vi "Construct LV Version String.vi"(8 "error in (no error)":errorcluster) -> (0 "error out":errorcluster, 3 "LabVIEW Version":string)   [LabVIEW 2014]
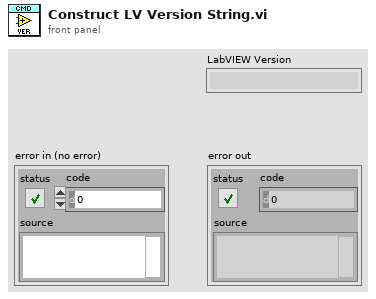
[diagram p1: front panel]
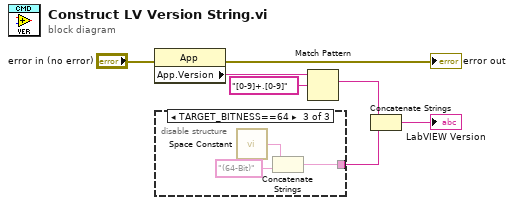
[diagram p0: block diagram]
diagram:
  n1 = property class="App"(error in="error in (no error)") -> (error out=→"error out":errorcluster, "App.Version"=w7:string)  [unwired: 1 in, 1 out]
  n2 = disable-structure shown="TARGET_BITNESS==64" {
    disable-tunnel: [_ _ w9] -> w4
    frame condition #0 {
    }
    frame condition #1 (active) {
    }
    frame condition #2 {
      n3 = call <vilib>:"Space Constant.vi"() -> ("String"=w8:string)
      n4 = Concatenate Strings(w8, "(64-Bit)" ("regular expression")) -> (w9:string)
    }
  }
  n5 = Match Pattern(string=w7, regular expression="[0-9]+.[0-9]") -> (match substring=w5:string)  [unwired: 1 in, 3 out]
  n6 = Concatenate Strings(w5, w4) -> (→"LabVIEW Version":string)
